vi "ResetTimer.vi"(8 "error in (no error)":errorcluster, 11 "Model in":refnum<class "Model.lvclass">) -> (0 "error out":errorcluster, 3 "Model out":refnum<class "Model.lvclass">)   [LabVIEW 2016, in "Model.lvclass"]
uses:
  Model.lvclass
  Model.lvclass/Model.ctl
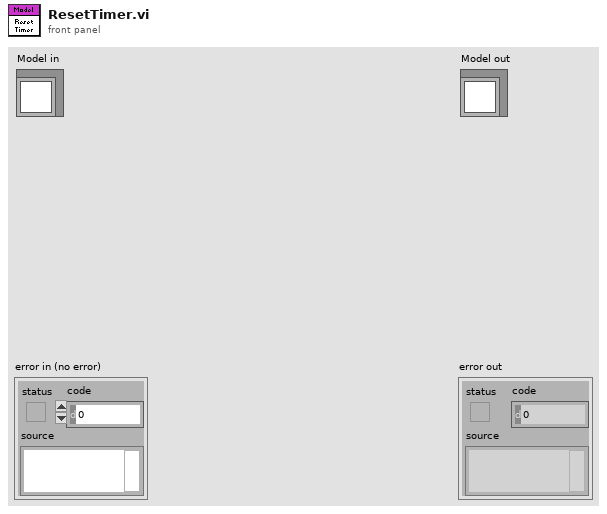
[diagram p1: front panel]
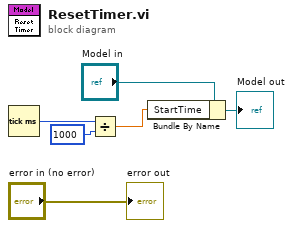
[diagram p0: block diagram]
diagram:
  n1 = Tick Count (ms)() -> (millisecond timer value=w3:u32)
  n2 = Divide(x=w3, y=u32 1000) -> (x/y=w1:dbl)
  n3 = Bundle By Name(cluster="Model in", "StartTime"=w1) -> (→"Model out":refnum<class "Model.lvclass">)
  "error out" <- "error in (no error)"
